vi "MakeAProfileJK.vi"(0 "image in":u8[][](array[numeric]), 1 "Rsin(phi)[Q]":dbl[][][](array[numeric]), 2 "angularbinlengths":i32[](array[numeric]), 5 "# Radial bins":u32, 7 "radial bins/pixel":dbl=32.0, 9 "window":dbl[](array[numeric]), 11 "error in (no error) 2":errorcluster, 12 "Rcos(phi)[Q]":dbl[][][](array[numeric])) -> (6 "radial profile":dbl[](array[numeric]), 10 "xy-out 1":dbl[](array[numeric]), 15 "error in (no error) 3":errorcluster)   [LabVIEW 2011, in "OfflineTracker.lvlib"]
doc: "This vi makes a radial profile around a center point from an image. points are from averaged circles via 4-point interpolated points. Each circle is mapped at 2pi.R points, where R is half the ROI sizes. JacobKers09"
uses:
  OfflineTracker.lvlib
panel:
  in  "stripe halfwidth":i8=9
  out "Bead":u8[][](graph)
  out "PreTrak XY Coordinates":dbl[](array[numeric]) format="%.2f"
  out "Position Correction":dbl[](array[numeric])
  out "COM Position (pixels)":dbl[](array[numeric])
  out "Intensity Graph":u8[][](graph)
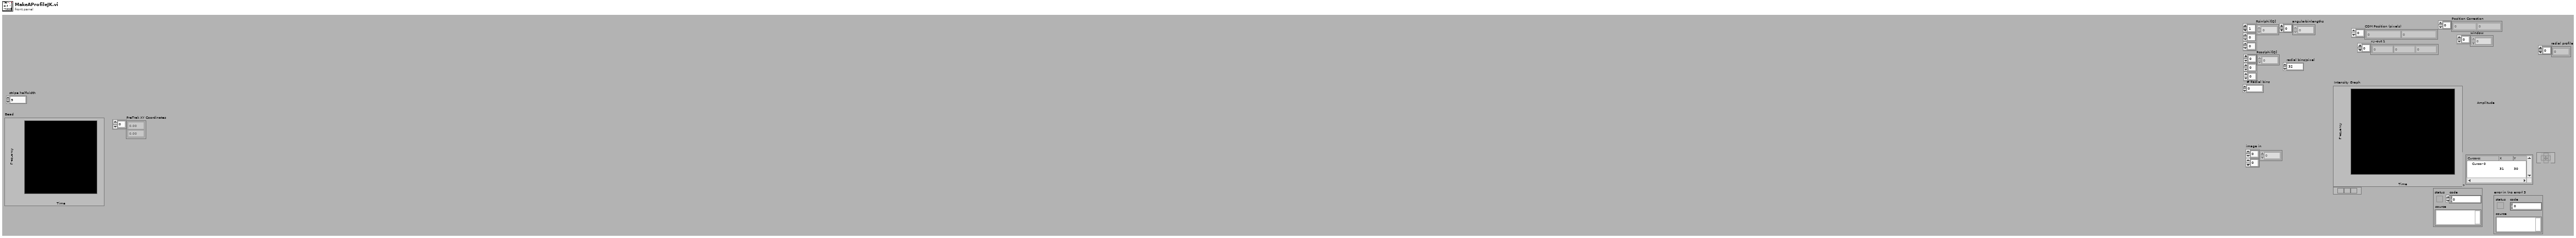
[diagram p1: front panel]
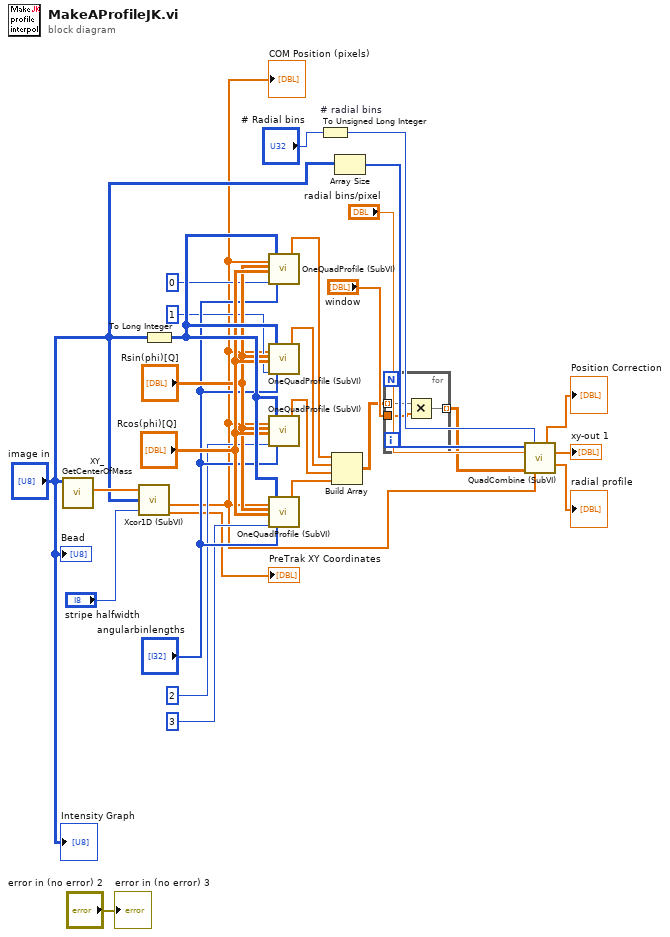
[diagram p0: block diagram]
diagram:
  n1 = call "XY_GetCenterOfMass.vi"("Image in"="image in") -> ("corner-based Coordinates (pix)"=w6:dbl[])  [unwired: 9 out]
  n2 = call "Xcor1D (SubVI).vi"("corner-based Coordinates (pix)"=w6, "Original Data"="image in", "stripe halfwidth"="stripe halfwidth") -> ("corner-based coordinates"=w4:dbl[], "center-based coordinates"=→"PreTrak XY Coordinates":dbl[])  [unwired: 3 in]
  "COM Position (pixels)" <- w4
  n3 = To Long Integer(number="image in") -> (32bit integer=w27:i32[][])
  n4 = call "OneQuadProfile (SubVI).vi"("corner-based \ncoordinates (pix)"=w4, "Rsin(phi)[Q]"="Rsin(phi)[Q]", "Rcos(phi)[Q]"="Rcos(phi)[Q]", "Quadrant?"=0 ("Numeric"), "Image"=w27, "lengths"="angularbinlengths") -> ("profile"=w13:dbl[])  [unwired: 3 in, 10 out]
  n5 = call "OneQuadProfile (SubVI).vi"("corner-based \ncoordinates (pix)"=w4, "Rsin(phi)[Q]"="Rsin(phi)[Q]", "Rcos(phi)[Q]"="Rcos(phi)[Q]", "Quadrant?"=1 ("Numeric"), "Image"=w27, "lengths"="angularbinlengths") -> ("profile"=w17:dbl[])  [unwired: 3 in, 10 out]
  n6 = call "OneQuadProfile (SubVI).vi"("corner-based \ncoordinates (pix)"=w4, "Rsin(phi)[Q]"="Rsin(phi)[Q]", "Rcos(phi)[Q]"="Rcos(phi)[Q]", "Quadrant?"=2 ("Numeric"), "Image"=w27, "lengths"="angularbinlengths") -> ("profile"=w14:dbl[])  [unwired: 3 in, 10 out]
  n7 = call "OneQuadProfile (SubVI).vi"("corner-based \ncoordinates (pix)"=w4, "Rsin(phi)[Q]"="Rsin(phi)[Q]", "Rcos(phi)[Q]"="Rcos(phi)[Q]", "Quadrant?"=3 ("Numeric"), "Image"=w27, "lengths"="angularbinlengths") -> ("profile"=w12:dbl[])  [unwired: 13 in]
  n8 = To Unsigned Long Integer "# radial bins"(number="# Radial bins") -> (unsigned 32bit integer=w11:u32)
  n9 = Build Array(w13, w17, w14, w12) -> (w2:dbl[][])
  n10 = Array Size(array="image in") -> (size(s)=w10:i32[])
  n11 = for {
    tunnel: w2 -> [w31] mode=indexing
    tunnel: [w30] -> w1 mode=indexing
    tunnel: "window" -> [w29]
    n12 = Multiply(x=w31, y=w29) -> (x*y=w30:dbl[])
  }
  n13 = call "QuadCombine (SubVI).vi"("roi"=w10, "# of radial bins"=w11, "radial bins/pixel"="radial bins/pixel", "profiles"=w1, "pre-xy (pixels)"=w4) -> ("Position Correction"=→"Position Correction":dbl[], "Position (pixels)"=→"xy-out 1":dbl[], "radial profile"=→"radial profile":dbl[])  [unwired: 1 in, 7 out]
  "error in (no error) 3" <- "error in (no error) 2"
  "Intensity Graph" <- "image in"
  "Bead" <- "image in"
